vi "Untitled 8.vi"() -> ()   [LabVIEW 2015]
uses:
  <vilib>/measure/NI_MAPro.lvlib
panel:
  out "String 2":string="Establecer las entradas a los\nvalores deseados y seleccionar\nuna formula"
  in  "offset":dbl format="%0.2p"
  in  "reset signal":bool
  in  "amplitude":dbl=1.0 format="%0.2p"
  in  "frequency":dbl=10.0 format="%0.2p"
  in  "String":string
  out "Numeric":dbl
  in  "Ring":u16(ring) items=["Usuario", "Pregrabado 2", "Pregrabado 1"]
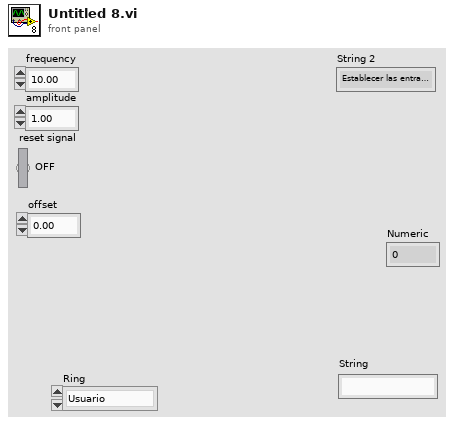
[diagram p1: front panel]
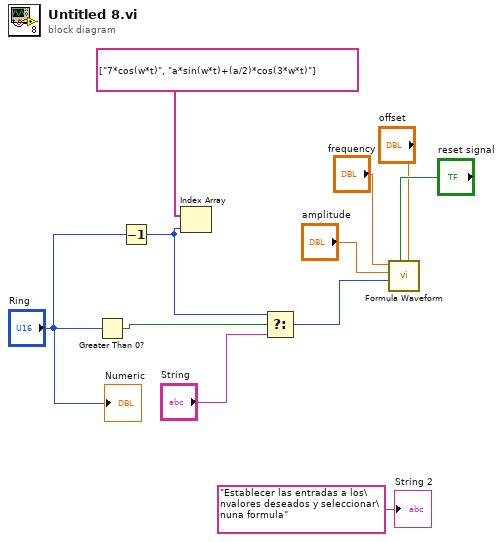
[diagram p0: block diagram]
diagram:
  n1 = Greater Than 0?(x="Ring") -> (x > 0?=w8:bool)
  n2 = Decrement(x="Ring") -> (x-1=w9:u16)
  n3 = Index Array(array=string[] ["7*cos(w*t)", "a*sin(w*t)+(a/2)*cos(3*w*t)"], index=w9) -> ()  [unwired: 1 out]
  n4 = Select(t=w9, s=w8, f="String") -> (s? t:f=w5:u16)
  n5 = call <vilib>:"Formula Waveform.vi"("offset"="offset", "reset signal"="reset signal", "formula"=w5, "amplitude"="amplitude", "frequency"="frequency") -> ()  [unwired: 5 in, 2 out]
  "Numeric" <- "Ring"
  "String 2" <- "Establecer las entradas a los\nvalores deseados y seleccionar\nuna formula"
